vi "Normalize HMI.vi"(8 "error in (no error)":errorcluster, 10 "Steering Frame in":T4, 11 "Device in":T1={"device ID"=refnum, "Device Name"="Logitech Extreme 3D", "axis info"={"X axis"=[], "Y axis"=[], "Z axis"=[], "X axis rotation"=[], "Y axis rotation"=[], "Z axis rotation"=[], "U axis"=[], "V axis"=[]}}) -> (0 "error out":errorcluster, 2 "Steering Frame out":T4, 3 "Device Out":T1={"device ID"=refnum, "Device Name"="Logitech Extreme 3D", "axis info"={"X axis"=[], "Y axis"=[], "Z axis"=[], "X axis rotation"=[], "Y axis rotation"=[], "Z axis rotation"=[], "U axis"=[], "V axis"=[]}})   [LabVIEW 2012]
uses:
  <vilib>/robotics/Steering/Class Type Definitions/Mecanum Steering Frame.ctl
  <vilib>/robotics/Steering/Mecanum Steering Frame/NI_Robotics_Mecanum Steering Frame.lvclass
  <vilib>/robotics/Steering/Class Type Definitions/Differential Steering Frame.ctl
  <vilib>/robotics/Steering/Differential Steering Frame/NI_Robotics_Differential Steering Frame.lvclass
  <vilib>/Utility/inputDevices.llb/joystickAcquire.vi
  <vilib>/robotics/Steering/Steering Frame/Apply Steering Frame Velocity to Wheels.vi
  <vilib>/robotics/Steering/Steering Frame/NI_Robotics_Steering Frame.lvclass
  <vilib>/robotics/Steering/Class Type Definitions/NI_Robotics_Steering Class Types.lvlib
panel:
  out "axis info":T5
  out "direction info":T6
  out "button info":T7
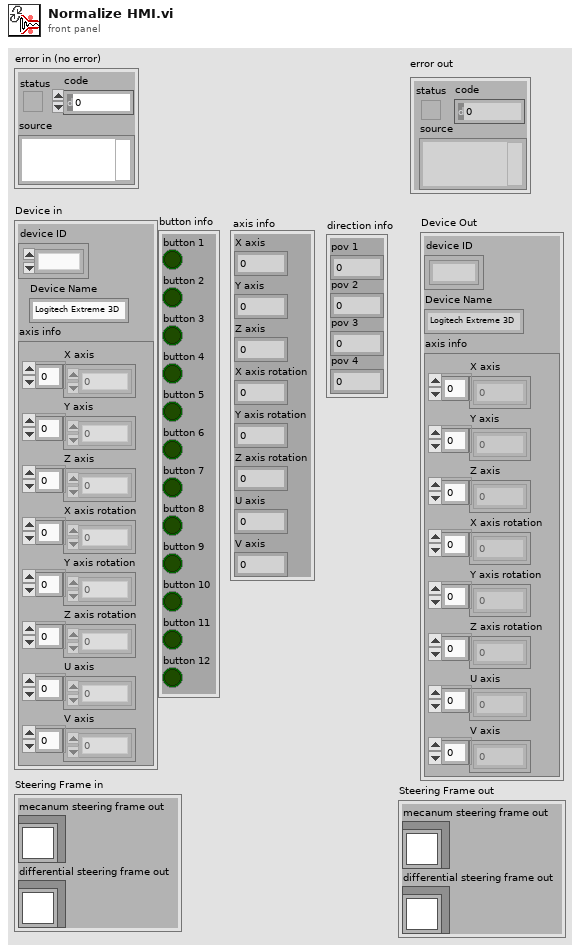
[diagram p1: front panel]
types:
  T1 = cluster{"device ID":refnum<k1>, "Device Name":string, "axis info":cluster{"X axis":dbl[], "Y axis":dbl[], "Z axis":dbl[], "X axis rotation":dbl[], "Y axis rotation":dbl[], "Z axis rotation":dbl[], "U axis":dbl[], "V axis":dbl[]}}
  T2 = typedef "NI_Robotics_Steering Class Types.lvlib/Mecanum Steering Frame.ctl" = refnum<class "NI_Robotics_Mecanum Steering Frame.lvclass">
  T3 = typedef "NI_Robotics_Steering Class Types.lvlib/Differential Steering Frame.ctl" = refnum<class "NI_Robotics_Differential Steering Frame.lvclass">
  T4 = cluster{"mecanum steering frame out":T2, "differential steering frame out":T3}
  T5 = cluster{"X axis":i32, "Y axis":i32, "Z axis":i32, "X axis rotation":i32, "Y axis rotation":i32, "Z axis rotation":i32, "U axis":i32, "V axis":i32}
  T6 = cluster{"pov 1":i32, "pov 2":i32, "pov 3":i32, "pov 4":i32}
  T7 = cluster{"button 1":bool, "button 2":bool, "button 3":bool, "button 4":bool, "button 5":bool, "button 6":bool, "button 7":bool, "button 8":bool, "button 9":bool, "button 10":bool, "button 11":bool, "button 12":bool, "button 13":bool, "button 14":bool, "button 15":bool, "button 16":bool, "button 17":bool, "button 18":bool, "button 19":bool, "button 20":bool, "button 21":bool, "button 22":bool, "button 23":bool, "button 24":bool, "button 25":bool, "button 26":bool, "button 27":bool, "button 28":bool, "button 29":bool, "button 30":bool, "button 31":bool, "button 32":bool}
  T8 = cluster{"X axis":dbl, "Y axis":dbl, "Z axis":dbl, "X axis rotation":dbl, "Y axis rotation":dbl, "Z axis rotation":dbl, "U axis":dbl, "V axis":dbl}
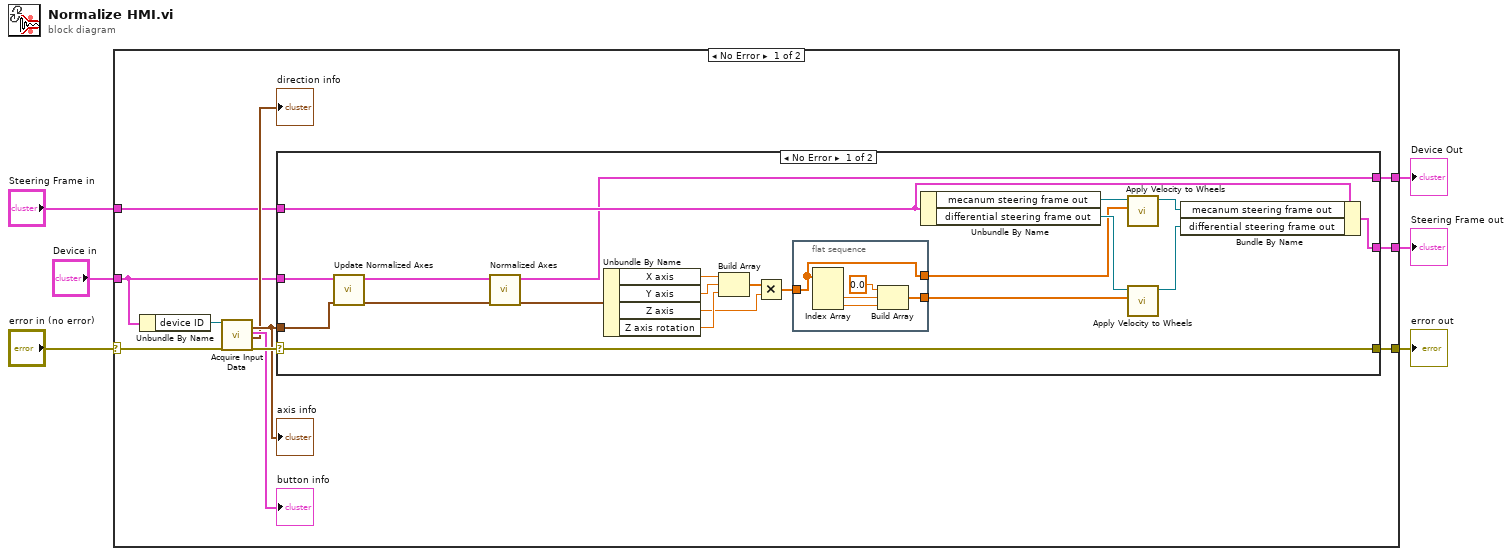
[diagram p0: block diagram]
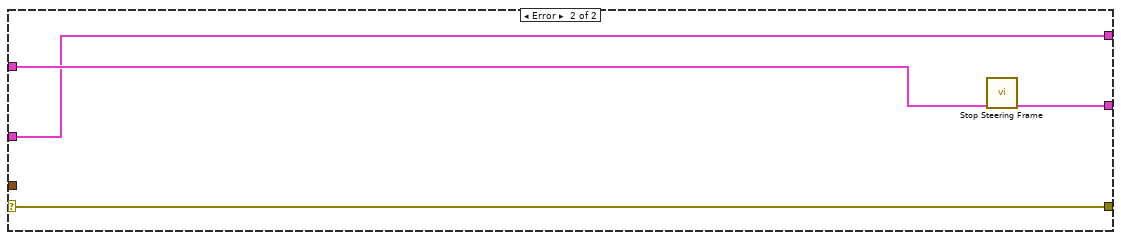
[diagram p2: hidden frame]
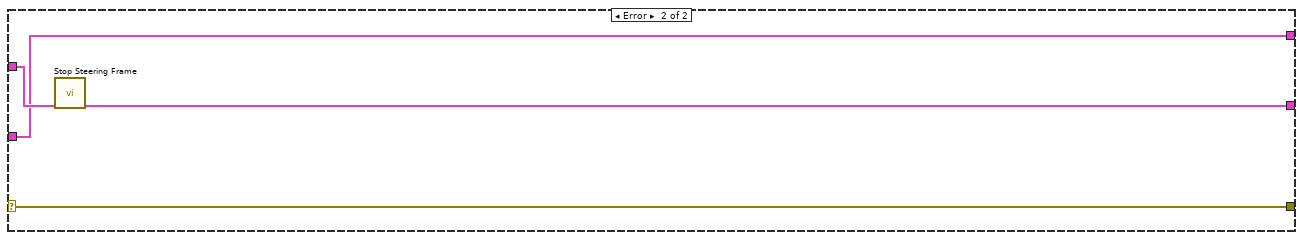
[diagram p3: hidden frame]
diagram:
  n1 = case shown="No Error" "error in (no error)" {
    selector: "error in (no error)" -> [w9 w49]
    tunnel: [w8 w49] -> w6
    tunnel: "Device in" -> [w12 w48]
    tunnel: "Steering Frame in" -> [w11 w51]
    tunnel: [w10 w50] -> w2
    tunnel: [w7 w48] -> w1
    frame No Error {
      n2 = Unbundle By Name(w12) -> ("device ID"=w16:refnum<k1>)
      n3 = call-poly <vilib>:"Acquire Input Data.vi"("device ID"=w16, "error in (no error)"=w9) -> ("axis info"=w14:T5, "button info"=→"button info":T7, "direction info"=→"direction info":T6, "error out"=w17:errorcluster)  [unwired: 13 in, 1 out]
      "axis info" <- w14
      n4 = case shown="No Error" w17 {
        selector: w17 -> [w36 w45]
        tunnel: w14 -> [w22 _]
        tunnel: w12 -> [w20 w44]
        tunnel: w11 -> [w38 w47]
        tunnel: [w37 w46] -> w10
        tunnel: [w36 w45] -> w8
        tunnel: [w18 w44] -> w7
        frame No Error {
          n5 = call "Update Normalized Axes.vi"("axis in"=w22, "Device in"=w20) -> ("axis out"=w21:T5, "Device out"=w19:T1)  [unwired: 8 in]
          n6 = call "Normalized Axes.vi"("axis in"=w21, "Device in"=w19) -> ("axis out"=w33:T8, "Device out"=w18:T1)  [unwired: 8 in]
          n7 = Unbundle By Name(w33) -> ("X axis"=w34:dbl, "Y axis"=w35:dbl, "Z axis"=w26:dbl, "Z axis rotation"=w30:dbl)
          n8 = Build Array(w34, w35, w30) -> (w23:dbl[])
          n9 = Multiply(x=w23, y=w26) -> (x*y=w25:dbl[])
          n10 = flat-sequence {
            tunnel: [w43] -> w29
            tunnel: w25 -> [w40]
            tunnel: [w40] -> w24
            frame #0 {
              n11 = Index Array(array=w40) -> (element #2=w41:dbl, element #3=w39:dbl)  [unwired: 3 in, 1 out]
              n12 = Build Array(0.0 ("element"), w41, w39) -> (w43:dbl[])
            }
          }
          n13 = Unbundle By Name(w38) -> ("mecanum steering frame out"=w32:T2, "differential steering frame out"=w31:T3)
          n14 = call-poly <vilib>:"Apply Velocity to Wheels.vi"("steering frame velocity"=w24, "steering frame in"=w32) -> ("steering frame out"=w28:T2)  [unwired: 6 in, 3 out]
          n15 = call-poly <vilib>:"Apply Velocity to Wheels.vi"("steering frame velocity"=w29, "steering frame in"=w31) -> ("steering frame out"=w27:T3)  [unwired: 6 in, 3 out]
          n16 = Bundle By Name(cluster=w38, "mecanum steering frame out"=w28, "differential steering frame out"=w27) -> (w37:T4)
        }
        frame Error {
          n17 = call "Stop Steering Frame.vi"("Steering Frame in"=w47) -> ("Steering Frame out"=w46:T4)  [unwired: 10 in]
        }
      }
    }
    frame Error {
      n18 = call "Stop Steering Frame.vi"("Steering Frame in"=w51) -> ("Steering Frame out"=w50:T4)  [unwired: 10 in]
    }
  }
  "error out" <- w6
  "Steering Frame out" <- w2
  "Device Out" <- w1
